vi "write_intercept_init.vi"(8 "error in (no error)":errorcluster, 10 "intercept_init":dbl[](array[numeric]), 11 "SGDClassifier in":refnum<class "SGDClassifier.lvclass">) -> (0 "error out":errorcluster, 3 "SGDClassifier out":refnum<class "SGDClassifier.lvclass">)   [LabVIEW 2020, in "SGDClassifier.lvclass"]
uses:
  SGDClassifier.lvclass
  SGDClassifier.lvclass/SGDClassifier.ctl
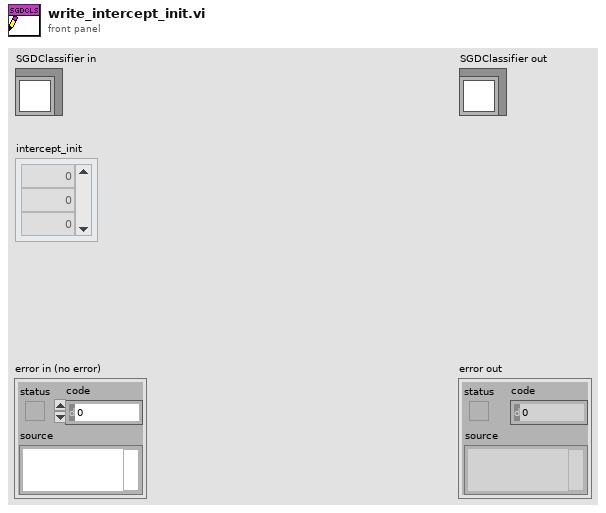
[diagram p1: front panel]
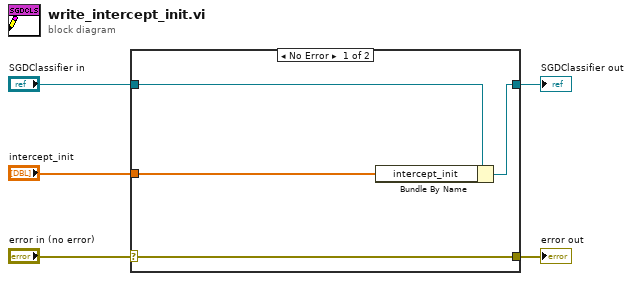
[diagram p0: block diagram]
diagram:
  n1 = case shown="No Error" "error in (no error)" {
    selector: "error in (no error)" -> [w9 w10]
    tunnel: [w9 w10] -> w4
    tunnel: [w7 w11] -> w2
    tunnel: "SGDClassifier in" -> [w8 w11]
    tunnel: "intercept_init" -> [w6 _]
    frame No Error {
      n2 = Bundle By Name(cluster=w8, "intercept_init"=w6) -> (w7:refnum<class "SGDClassifier.lvclass">)
    }
    frame Error {
    }
  }
  "error out" <- w4
  "SGDClassifier out" <- w2
